vi "pp2_log_error.vi"(6 "error in (no error)":errorcluster, 9 "queue in":refnum<queue>) -> (0 "error out":errorcluster, 3 "queue out":refnum<queue>)   [LabVIEW 2013]
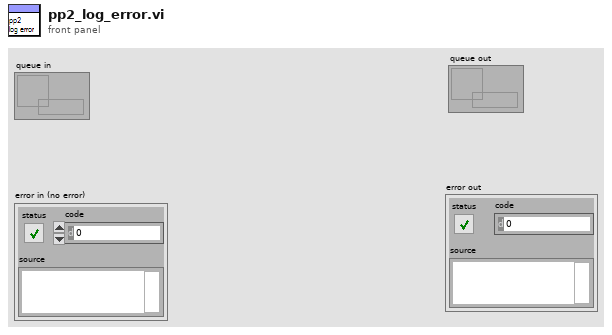
[diagram p1: front panel]
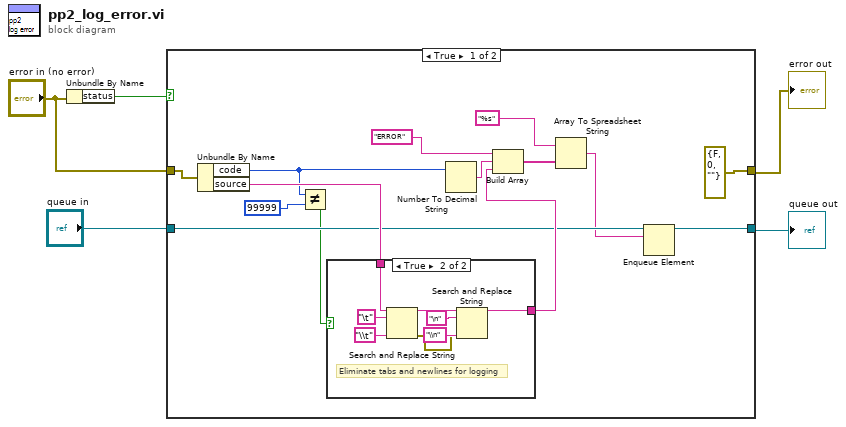
[diagram p0: block diagram]
diagram:
  n1 = Unbundle By Name("error in (no error)") -> ("status"=w5:bool)
  n2 = case shown="True" w5 {
    tunnel: "error in (no error)" -> [w19 w29]
    tunnel: "queue in" -> [w11 w30]
    tunnel: [w10 w30] -> w1
    tunnel: [errorcluster {"status"=FALSE, "code"=0, "source"=""} ("error in (no error)") w29] -> w3
    frame True {
      n3 = Unbundle By Name(w19) -> ("code"=w7:i32, "source"=w13:string)
      n4 = Not Equal?(x=w7, y=99999 ("code")) -> (x != y?=w6:bool)
      n5 = case shown="True" w6 {
        tunnel: w13 -> [w20 w28]
        tunnel: [w20 w21] -> w12
        frame False {
        }
        frame True {
          # "Eliminate tabs and newlines for logging"
          n6 = Search and Replace String(input string=w28, search string="\t", replace string="\\t" ("replace string (\"\")")) -> (result string=w23:string, error out=w22:errorcluster)  [unwired: 5 in, 2 out]
          n7 = Search and Replace String(input string=w23, search string="\n", replace string="\\n" ("replace string (\"\")"), error in=w22) -> (result string=w21:string)  [unwired: 4 in, 3 out]
        }
      }
      n8 = Number To Decimal String(number=w7) -> (decimal integer string=w17:string)  [unwired: 1 in]
      n9 = Build Array("ERROR" ("element"), w17, w12) -> (w15:string[])
      n10 = Array To Spreadsheet String(array=w15, 3:"%s" ("format string")) -> (spreadsheet string=w9:string)  [unwired: 1 in]
      n11 = Enqueue Element(queue=w11, element=w9) -> (queue out=w10:refnum<queue>)  [unwired: 2 in, 2 out]
    }
    frame False {
    }
  }
  "error out" <- w3
  "queue out" <- w1
